vi "SRV_Wait_msec.vi"(0 "Wait time in msec":string="100", 2 "SuperPro":T1) -> (4 "SuperPro":T1)   [LabVIEW 2009]
doc: "Waits for a specific number of msec. By default it uses Timer3. If nothing is wired into the string value then it uses the integer (use the string to specify another variable)."
uses:
  <userlib>/SuperPro/OpCodes/_SubVIs/SuperProControl.ctl
panel:
  # "This LabVIEW item is deprecated.\n\nIt is believed to be unused and will be removed in a future version of SRV."
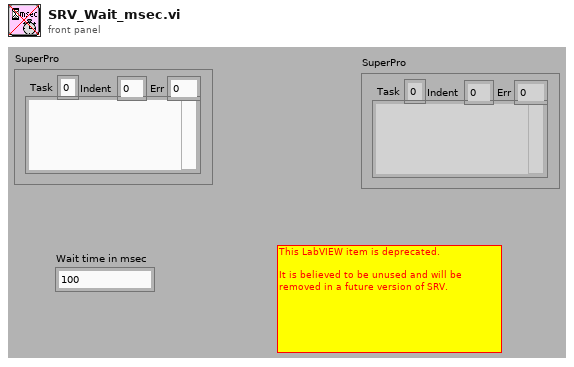
[diagram p1: front panel]
types:
  T1 = typedef "SuperProControl.ctl" = cluster{"Task":i32, "Indent":i32, "Err":i32, "ASM":string}
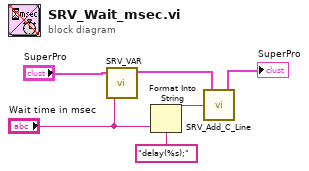
[diagram p0: block diagram]
diagram:
  n1 = call "SRV_VAR.vi"("SuperPro in"="SuperPro", "Name"="Wait time in msec") -> ("SuperPro out"=w2:T1)  [unwired: 1 in, 3 out]
  n2 = Format Into String(format string="delay(%s);", "Wait time in msec") -> (resulting string=w5:string)  [unwired: 2 in, 1 out]
  n3 = call "SRV_Add_C_Line.vi"("C String"=w5, "SuperPro in"=w2) -> ("SuperPro out"=→"SuperPro":T1)  [unwired: 3 in]
